vi "Mini Bach random sampling_R_sub.vi"(0 "Mini Bach No.":i32, 1 "MNIST Input":i32[][](array[numeric])) -> (2 "MNIST Random Output":i32[][](array[numeric]), 3 "MNIST No.Row":i32[](array[numeric]), 4 "MNIST Num":i32[](array[numeric]))   [LabVIEW 2021]
uses:
  <vilib>/numeric/Random Number (Range) I64.vi
  <vilib>/numeric/sub_Random U32.vi
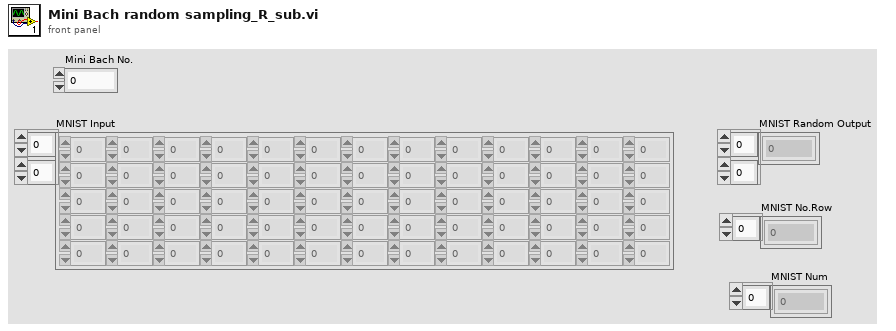
[diagram p1: front panel]
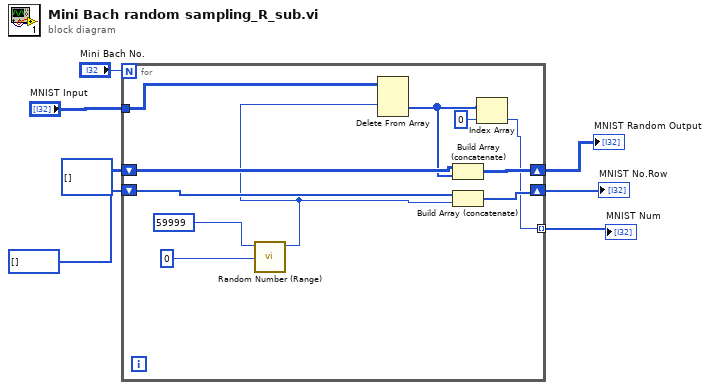
[diagram p0: block diagram]
diagram:
  n1 = for {
    N: "Mini Bach No." -> [_]
    shift-right: [w18] -> w6
    shift-left: i32[][] [] -> [w17]
    shift-right: [w16] -> w5
    shift-left: i32[] [] -> [w15]
    tunnel: "MNIST Input" -> [w14]
    tunnel: [w8] -> w1 mode=indexing
    n2 = call-poly <vilib>:"Random Number (Range).vi"("lower bound (-100)"=i64 0, "upper bound (100)"=i64 59999) -> ("number"=w11:i64)  [unwired: 9 in]
    n3 = Delete From Array(array=w14, index (row)=w11) -> (deleted portion=w10:i32[])  [unwired: 2 in, 1 out]
    n4 = Build Array (concatenate)(w17, w10) -> (w18:i32[][])
    n5 = Build Array (concatenate)(w15, w11) -> (w16:i64[])
    n6 = Index Array(array=w10, index=0 ("인덱스")) -> (element=w8:i32)
  }
  "MNIST Random Output" <- w6
  "MNIST No.Row" <- w5
  "MNIST Num" <- w1
